vi "test_Script_664_custom_device.vi"(0 "TestCase in":refnum<class "Scripting.lvclass">, 3 "error in":errorcluster) -> (7 "TestCase out":refnum<class "Scripting.lvclass">, 10 "error out":errorcluster)   [LabVIEW 2020, in "Scripting.lvclass"]
uses:
  Scripting.lvclass
  C:/Program Files (x86)/National Instruments/LabVIEW 2020/vi.lib/NI/VeriStand Custom Device Testing Tools/VeriStandScriptingTestCase/VeriStandScriptingTestCase.lvclass
  <vilib>/NI/VeriStand Custom Device Testing Tools/VeriStandScriptingTestCase/VeriStandScriptingTestCase.lvclass/VeriStandScriptingTestCase.ctl
  <vilib>/NI/VeriStand Custom Device Testing Tools/VeriStandScriptingTestCase/Read Target.vi
  NationalInstruments.VeriStand.SystemDefinitionAPI
  Scripting/AIM ARINC 664 Scripting.lvlib
  <vilib>/addons/_JKI Toolkits/VI Tester/TestCase.llb/TestCase.lvclass
  C:/Program Files (x86)/National Instruments/LabVIEW 2020/vi.lib/addons/_JKI Toolkits/VI Tester/TestCase.llb/TestCase.lvclass
  C:/repos/niveristand-aim-arinc664-custom-device/Source/Custom Device Support/Tests/Unit/Scripting/Scripting.lvclass
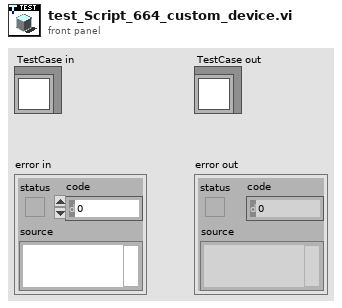
[diagram p1: front panel]
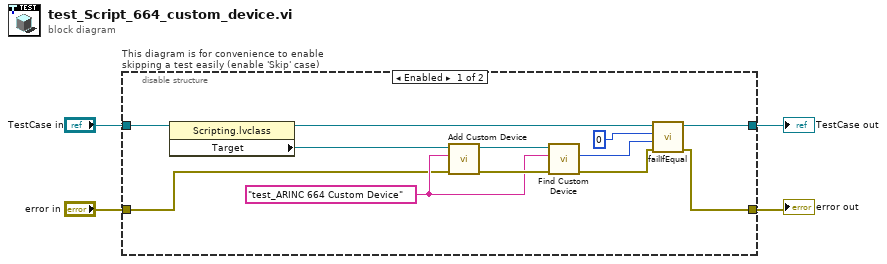
[diagram p0: block diagram]
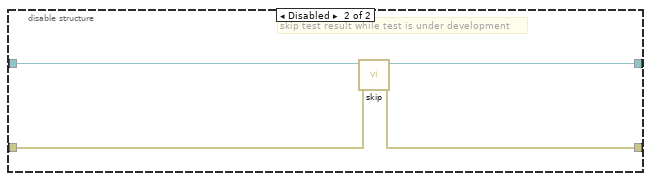
[diagram p2: hidden frame]
diagram:
  n1 = disable-structure "This diagram is for convenience to enable skipping a test easily (enable 'Skip' case)" shown="Enabled" {
    disable-tunnel: "TestCase in" -> [w6 w20]
    disable-tunnel: [w10 w18] -> w1
    disable-tunnel: [w13 w19] -> w3
    disable-tunnel: "error in" -> [w5 w17]
    frame Enabled {
      w11 = "test_ARINC 664 Custom Device" ("name")
      n2 = property class="Scripting.lvclass"(reference=w6) -> (reference out=w7:refnum<class "Scripting.lvclass">, "Target"=w8:refnum<k24>)  [unwired: 1 in, 1 out]
      n3 = call "Add Custom Device.vi"("error in"=w5, "name"=w11, "target in"=w8) -> ("error out"=w16:errorcluster, "target out"=w15:refnum<k24>)  [unwired: 6 in, 1 out]
      n4 = call "Find Custom Device.vi"("error in"=w16, "name"=w11, "target in"=w15) -> ("error out"=w14:errorcluster, "custom device"=w12:u64)  [unwired: 6 in, 1 out]
      n5 = call-dynamic "failIfEqual.vi"("error in (no error)"=w14, "y"=w12, "x"=u64 0 ("custom device"), "TestCase in"=w7) -> ("error out"=w13:errorcluster, "TestCase out"=w10:refnum<class "Scripting.lvclass">)  [unwired: 6 in]
    }
    frame Disabled {
      # "skip test result while test is under development"
      n6 = call <vilib>:"skip.vi"("error in (no error)"=w17, "TestCase in"=w20) -> ("error out"=w19:errorcluster, "TestCase out"=w18:refnum<class "Scripting.lvclass">)  [unwired: 8 in]
    }
  }
  "error out" <- w3
  "TestCase out" <- w1
